vi "215.Recipe Loop Load (Sub VI).vi"(0 "VISA Gilson":refnum<visa-resource-name>, 1 "VISA Multi-position Valve":refnum<visa-resource-name>, 2 "VISA Isolation Valve":refnum<visa-resource-name>, 3 "Y Position List":u16[](array[numeric]), 4 "Volume List":u16[](array[numeric]), 5 "error in (no error)":errorcluster, 6 "X Position List":u16[](array[numeric]), 7 "Flush Position":u16=1, 8 "Flush Volume":u16=1000, 9 "Reactor Position":u16=2, 10 "Syringe Cycle (ms)":u16=15000, 12 "Needle Sample Position":u16=1000) -> (14 "VISA Gilson Out":refnum<visa-resource-name>, 15 "VISA Multi-position Valve Out":refnum<visa-resource-name>, 19 "error out":errorcluster)   [LabVIEW 2020]
uses:
  <instrlib>/rheodyne/rheodyne.lvlib
panel:
  # "The vectors refers to the reagent \"recipe\" for the reaction"
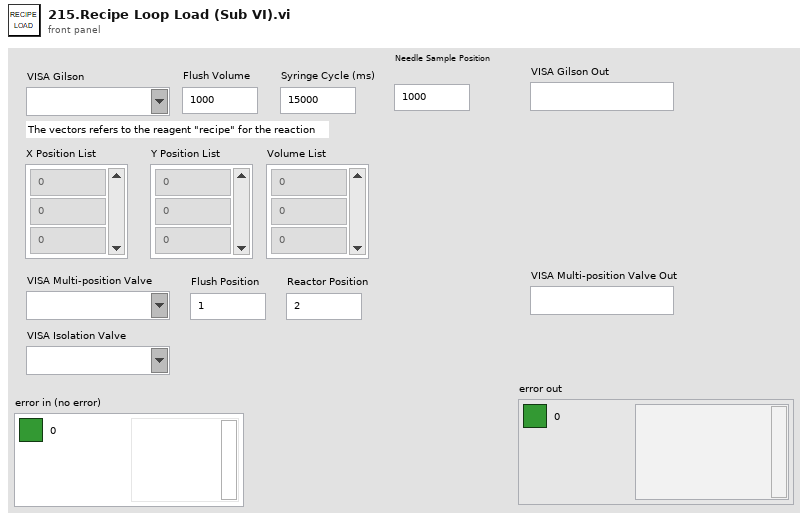
[diagram p1: front panel]
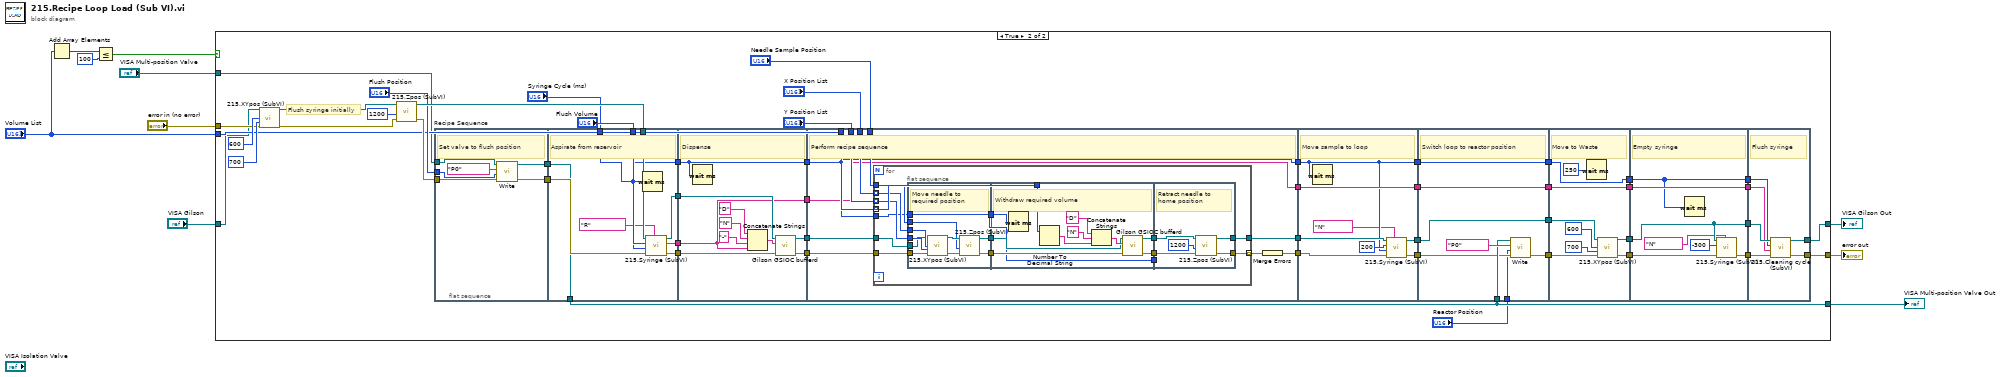
[diagram p0: block diagram]
diagram:
  n1 = Add Array Elements(numeric array="Volume List") -> (sum=w6:u16)
  n2 = Less Or Equal?(x=w6, y=u16 100) -> (x <= y?=w4:bool)
  n3 = case shown="True" w4 {
    tunnel: [w12 w31] -> w10
    tunnel: [w11 w30] -> w9
    tunnel: [w13 w28] -> w8
    tunnel: "Volume List" -> [_ w26]
    tunnel: "error in (no error)" -> [w12 w24]
    tunnel: "VISA Gilson" -> [w11 w23]
    tunnel: "VISA Multi-position Valve" -> [w13 w22]
    frame False {
    }
    frame True {
      # "Flush syringe initially"
      n4 = call "215.XYpos (SubVI).vi"("VISA resource name"=w23, "X"=600, "Y"=700, "error in (no error)"=w24) -> ("VISA Out"=w39:refnum<visa-resource-name>, "error out"=w40:errorcluster)  [unwired: 8 in, 2 out]
      n5 = call "215.Zpos (SubVI).vi"("error in (no error)"=w40, "Z"=1200, "VISA resource name"=w39) -> ("error out"=w33:errorcluster, "VISA Out"=w35:refnum<visa-resource-name>)  [unwired: 5 in, 2 out]
      n6 = flat-sequence "Recipe Sequence" {
        tunnel: w33 -> [w68]
        tunnel: w22 -> [w69]
        tunnel: "Flush Position" -> [w67]
        tunnel: [w66] -> w64
        tunnel: [w65] -> w63
        tunnel: "Flush Volume" -> [w79]
        tunnel: w35 -> [w78]
        tunnel: [w76] -> w62
        tunnel: [w75] -> w61
        tunnel: "Syringe Cycle (ms)" -> [w71]
        tunnel: [w71] -> w60
        tunnel: [w74] -> w59
        tunnel: w64 -> [w77]
        tunnel: w63 -> [w73]
        tunnel: [w73] -> w28
        tunnel: w62 -> [w85]
        tunnel: w61 -> [w84]
        tunnel: w60 -> [w89]
        tunnel: [w89] -> w57
        tunnel: w59 -> [w81]
        tunnel: [w82] -> w58
        tunnel: [w81] -> w56
        tunnel: [w80] -> w55
        tunnel: "X Position List" -> [w100]
        tunnel: "Y Position List" -> [w99]
        tunnel: w26 -> [w98]
        tunnel: w58 -> [w97]
        tunnel: "Needle Sample Position" -> [w96]
        tunnel: [w94] -> w54
        tunnel: [w93] -> w53
        tunnel: [w92] -> w52
        tunnel: w57 -> [w92]
        tunnel: [w91] -> w51
        tunnel: w56 -> [w91]
        tunnel: w55 -> [w90]
        tunnel: w54 -> [w142]
        tunnel: w53 -> [w147]
        tunnel: [w146] -> w50
        tunnel: [w141] -> w49
        tunnel: [w144] -> w48
        tunnel: w52 -> [w144]
        tunnel: [w148] -> w47
        tunnel: w51 -> [w148]
        tunnel: w50 -> [w156]
        tunnel: [w156] -> w46
        tunnel: w49 -> [w151]
        tunnel: [w150] -> w45
        tunnel: w48 -> [w155]
        tunnel: [w155] -> w44
        tunnel: w47 -> [w154]
        tunnel: [w154] -> w43
        tunnel: w28 -> [w152]
        tunnel: "Reactor Position" -> [w149]
        tunnel: w46 -> [w162]
        tunnel: w45 -> [w161]
        tunnel: [w160] -> w21
        tunnel: [w159] -> w19
        tunnel: [w158] -> w17
        tunnel: w44 -> [w158]
        tunnel: [w157] -> w15
        tunnel: w43 -> [w157]
        tunnel: w21 -> [w170]
        tunnel: [w170] -> w20
        tunnel: w19 -> [w169]
        tunnel: [w168] -> w18
        tunnel: w17 -> [w166]
        tunnel: [w166] -> w16
        tunnel: w15 -> [w172]
        tunnel: [w172] -> w14
        tunnel: w20 -> [w178]
        tunnel: w18 -> [w177]
        tunnel: w16 -> [w176]
        tunnel: w14 -> [w175]
        tunnel: [w174] -> w31
        tunnel: [w173] -> w30
        frame #0 {
          # "Set valve to flush position"
          n7 = call <instrlib>:"Write.vi"("error in (no error)"=w68, "Numeric"=w67, "Combo Box"="P0", "VISA resource name"=w69) -> ("error out"=w66:errorcluster, "VISA resource name 2"=w65:refnum<visa-resource-name>)  [unwired: 6 in]
        }
        frame #1 {
          # "Aspirate from reservoir"
          n8 = Wait (ms)(milliseconds to wait=w71) -> ()  [unwired: 1 out]
          n9 = call "215.Syringe (SubVI).vi"("Source"="R", "error in (no error)"=w77, "Syringe Cycle (ms)"=w71, "Flush Volume"=w79, "VISA Refnum in"=w78) -> ("error out"=w76:errorcluster, "String"=w74:string, "VISA Refnum out"=w75:refnum<visa-resource-name>)  [unwired: 4 in]
        }
        frame #2 {
          # "Dispense"
          n10 = Wait (ms)(milliseconds to wait=w89) -> ()  [unwired: 1 out]
          n11 = Concatenate Strings("D" ("string"), "N" ("string"), "-" ("string"), w81) -> (w83:string)
          n12 = call <instrlib>:"Gilson GSIOC bufferd.vi"("error in (no error)"=w85, "Bufferd command"=w83, "VISA resource name"=w84) -> ("error out"=w80:errorcluster, "VISA resource name out"=w82:refnum<visa-resource-name>)  [unwired: 6 in, 1 out]
        }
        frame #3 {
          # "Perform recipe sequence"
          n13 = for {
            tunnel: w100 -> [w111] mode=indexing
            tunnel: w99 -> [w110] mode=indexing
            tunnel: w98 -> [w115] mode=indexing
            tunnel: w97 -> [w109]
            tunnel: w90 -> [w108]
            tunnel: w96 -> [w107]
            tunnel: [w105] -> w95 mode=indexing
            tunnel: [w104] -> w93
            tunnel: w92 -> [w102]
            n14 = flat-sequence {
              tunnel: [w123] -> w114
              tunnel: [w122] -> w112
              tunnel: w108 -> [w121]
              tunnel: w111 -> [w120]
              tunnel: w110 -> [w119]
              tunnel: w109 -> [w118]
              tunnel: w107 -> [w117]
              tunnel: [w116] -> w103
              tunnel: w102 -> [w116]
              tunnel: w115 -> [w131]
              tunnel: w114 -> [w130]
              tunnel: [w129] -> w113
              tunnel: w112 -> [w128]
              tunnel: [w127] -> w106
              tunnel: w103 -> [w126]
              tunnel: [w126] -> w101
              tunnel: w113 -> [w139]
              tunnel: [w138] -> w104
              tunnel: w106 -> [w137]
              tunnel: [w136] -> w105
              tunnel: w101 -> [_]
              frame #0 {
                # "Move needle to required position"
                n15 = call "215.XYpos (SubVI).vi"("VISA resource name"=w118, "X"=w120, "Y"=w119, "error in (no error)"=w121) -> ("VISA Out"=w124:refnum<visa-resource-name>, "error out"=w125:errorcluster)  [unwired: 8 in, 2 out]
                n16 = call "215.Zpos (SubVI).vi"("error in (no error)"=w125, "Z"=w117, "VISA resource name"=w124) -> ("error out"=w122:errorcluster, "VISA Out"=w123:refnum<visa-resource-name>)  [unwired: 5 in, 2 out]
              }
              frame #1 {
                # "Withdraw required volume"
                n17 = Wait (ms)(milliseconds to wait=w126) -> ()  [unwired: 1 out]
                n18 = Number To Decimal String(number=w131) -> (decimal integer string=w132:string)  [unwired: 1 in]
                n19 = Concatenate Strings("D" ("string"), "N" ("string"), w132) -> (w133:string)
                n20 = call <instrlib>:"Gilson GSIOC bufferd.vi"("error in (no error)"=w128, "Bufferd command"=w133, "VISA resource name"=w130) -> ("error out"=w127:errorcluster, "VISA resource name out"=w129:refnum<visa-resource-name>)  [unwired: 6 in, 1 out]
              }
              frame #2 {
                # "Retract needle to home position"
                n21 = call "215.Zpos (SubVI).vi"("error in (no error)"=w137, "Z"=1200, "VISA resource name"=w139) -> ("error out"=w136:errorcluster, "VISA Out"=w138:refnum<visa-resource-name>)  [unwired: 5 in, 2 out]
              }
            }
          }
          n22 = Merge Errors(w95) -> (w94:errorcluster)
        }
        frame #4 {
          # "Move sample to loop"
          n23 = Wait (ms)(milliseconds to wait=w144) -> ()  [unwired: 1 out]
          n24 = call "215.Syringe (SubVI).vi"("Source"="N", "error in (no error)"=w142, "Syringe Cycle (ms)"=w144, "Flush Volume"=200, "VISA Refnum in"=w147) -> ("error out"=w141:errorcluster, "VISA Refnum out"=w146:refnum<visa-resource-name>)  [unwired: 4 in, 1 out]
        }
        frame #5 {
          # "Switch loop to reactor position"
          n25 = call <instrlib>:"Write.vi"("error in (no error)"=w151, "Numeric"=w149, "Combo Box"="P0", "VISA resource name"=w152) -> ("error out"=w150:errorcluster)  [unwired: 6 in, 1 out]
        }
        frame #6 {
          # "Move to Waste"
          n26 = Wait (ms)(milliseconds to wait=u32 250) -> ()  [unwired: 1 out]
          n27 = call "215.XYpos (SubVI).vi"("VISA resource name"=w162, "X"=600, "Y"=700, "error in (no error)"=w161) -> ("VISA Out"=w160:refnum<visa-resource-name>, "error out"=w159:errorcluster)  [unwired: 8 in, 2 out]
        }
        frame #7 {
          # "Empty syringe"
          n28 = Wait (ms)(milliseconds to wait=w166) -> ()  [unwired: 1 out]
          n29 = call "215.Syringe (SubVI).vi"("Source"="N", "error in (no error)"=w169, "Flush Volume"=-300, "VISA Refnum in"=w170) -> ("error out"=w168:errorcluster)  [unwired: 5 in, 2 out]
        }
        frame #8 {
          # "Flush syringe"
          n30 = call "215.Cleaning cycle (SubVI).vi"("error in (no error)"=w177, "Volumen (-1000 to 0)"=w175, "milliseconds to wait"=w176, "VISA Refnum in"=w178) -> ("error out"=w174:errorcluster, "VISA out"=w173:refnum<visa-resource-name>)  [unwired: 5 in, 1 out]
        }
      }
    }
  }
  "error out" <- w10
  "VISA Multi-position Valve Out" <- w8
  "VISA Gilson Out" <- w9
